vi "GetRegistrySecretKey.vi"(11 "Registry-SMO in":refnum<data-value>) -> (2 "SecretKey":string, 3 "Registry-SMO out":refnum<data-value>)   [LabVIEW 2013, in "Registry-SMO.lvclass"]
uses:
  Registry-SMO.lvclass
  Registry-SMO.lvclass/Registry-SMO.ctl
  Support/Attribute.Identity/Attribute.Identity.lvclass/Attribute.Identity.ctl
  Support/Attribute.Identity/Attribute.Identity.lvclass
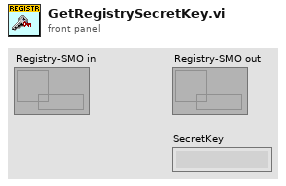
[diagram p1: front panel]
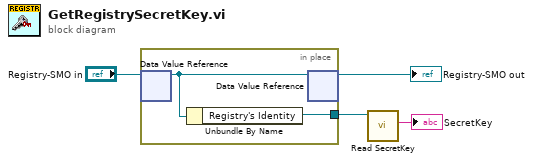
[diagram p0: block diagram]
diagram:
  n1 = in-place {
    in-place-border: [w5] -> w3
    n2 = in-place-dvr #1("Registry-SMO in") -> (w6:refnum<class "Registry-SMO.lvclass">)  [unwired: 1 out]
    n3 = Unbundle By Name(w6) -> ("Registry's Identity"=w5:refnum<class "Attribute.Identity.lvclass">)
    n4 = in-place-dvr #1(w6) -> (→"Registry-SMO out":refnum<data-value>)  [unwired: 1 out]
  }
  n5 = call "Read SecretKey.vi"("Attribute.Identity in"=w3) -> ("SecretKey"=→"SecretKey":string)  [unwired: 8 in, 2 out]
